vi "Reset Controls.vi"(8 "error in (no error)":errorcluster, 11 "Function UI in":refnum<class "Controller UI.lvclass">) -> (0 "error out":errorcluster, 3 "Function UI out":refnum<class "Controller UI.lvclass">)   [LabVIEW 2016, in "Controller UI.lvlib" / "Controller UI.lvclass"]
uses:
  <userlib>/Common Components/Controller UI/Controller UI.lvclass
  <userlib>/Common Components/User Interface/UI.lvclass
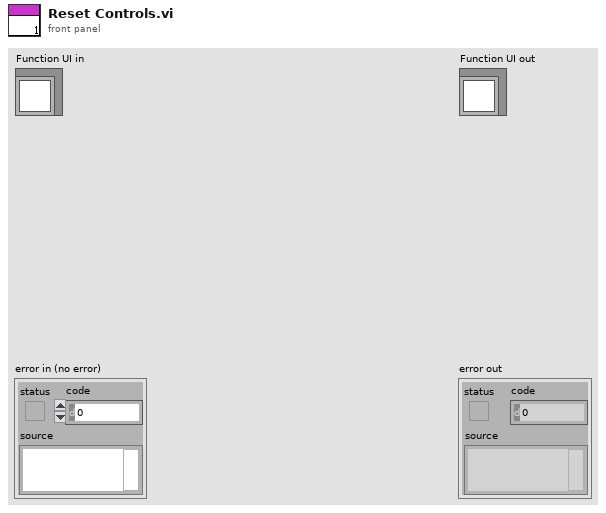
[diagram p1: front panel]
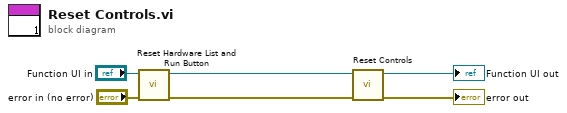
[diagram p0: block diagram]
diagram:
  n1 = call <userlib>:"Reset Hardware List and Run Button.vi"("error in (no error)"="error in (no error)", "Function UI in"="Function UI in") -> ("error out"=w2:errorcluster, "Function UI out"=w1:refnum<class "Controller UI.lvclass">)  [unwired: 8 in]
  n2 = call-parent "Reset Controls.vi"("error in (no error)"=w2, "UI in"=w1) -> ("error out"=→"error out":errorcluster, "UI out"=→"Function UI out":refnum<class "Controller UI.lvclass">)  [unwired: 8 in]
